vi "FPGA Read Sample.vi"(9 "Number samples\nafter trigger":i32, 10 "Number of Channels":i32, 11 "Timeout":i32) -> (0 "error out":errorcluster, 1 "Different Channel Count":bool, 2 "DMA FIFO Full":bool, 3 "Actual Loop Period (ticks)":u32)   [LabVIEW 2014]
uses:
  <vilib>/rvi/eio/common/nirviEmuClasses.ctl
  <vilib>/rvi/Emulation/niFpgaGetClockAttributes.vi
  <vilib>/rvi/Emulation/niFpgaSctlEmulationGetInTimedLoop.vi
  <vilib>/rvi/Emulation/niFpgaEmulationReportErrorSimple.vi
  FPGA Globals.vi
  <vilib>/rvi/eio/common/nirviEmuTemplateMethod_errors.vi
  <vilib>/rvi/interface/RandomDataEmulation/niFpgaRandomDataHandleErrors.vi
  <vilib>/rvi/Emulation/niFpgaProcessEmulError.vi
  <vilib>/rvi/Emulation/niFpgaCriticalErrorInLSC.vi
  <vilib>/eio/EIOGrowableMethodNode/genericMethod/EIOGrowableMethodNode.xnode
  <vilib>/rvi/eio/nirviEIOMethodImplementation/nirviEIOMethodImplementation.xnode
  <vilib>/rvi/eio/nirviErrorMerge/nirviErrorMerge.xnode
  <vilib>/rvi/DataTransferAndStorage/Container/XNode/niFpgaContainer.xnode
  <vilib>/rvi/interface/RandomDataEmulation/nirviRandomDataFpgaReadWriteTemplate.vi
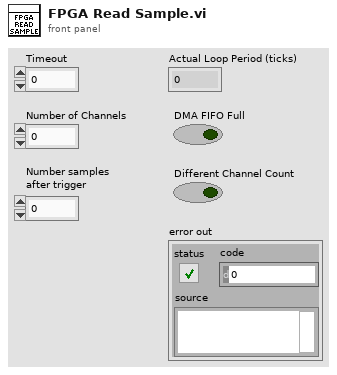
[diagram p1: front panel]
types:
  T1 = typedef "nirviEmuClasses.ctl" = enum16{"IO Read", "IO Write", "Method", "Property Read", "Property Write"}
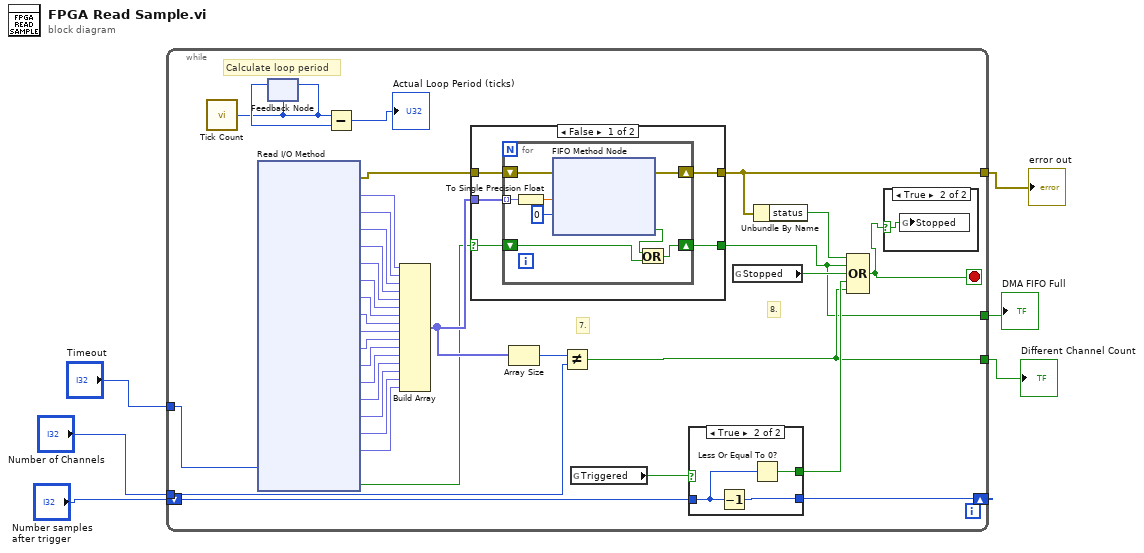
[diagram p0: block diagram]
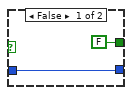
[diagram p3: hidden frame]
diagram:
  n1 = while {
    tunnel: [w41] -> w1
    tunnel: "Number of Channels" -> [w33]
    shift-right: [w30] -> _
    shift-left: "Number samples\nafter trigger" -> [w31]
    tunnel: [w26] -> w4
    tunnel: [w25] -> w5
    tunnel: "Timeout" -> [w23]
    stop <- w29 stop-if-true
    # "Calculate loop period"
    # "8."
    # "7."
    n2 = call "Tick Count"() -> ("Tick Count(Ticks)"=w35:u32)
    n3 = xnode "Read I/O Method"("Timeout"=w23) -> ("error out"=w40:errorcluster, "Mod2/AI0"=w24:fxp<+/-,24,5>, "Mod2/AI1"=w22:fxp<+/-,24,5>, "Mod2/AI2"=w21:fxp<+/-,24,5>, "Mod2/AI3"=w20:fxp<+/-,24,5>, "Mod2/AI4"=w19:fxp<+/-,24,5>, "Mod2/AI5"=w18:fxp<+/-,24,5>, "Mod2/AI6"=w17:fxp<+/-,24,5>, "Mod2/AI7"=w16:fxp<+/-,24,5>, "Mod2/AI8"=w15:fxp<+/-,24,5>, "Mod2/AI9"=w14:fxp<+/-,24,5>, "Mod2/AI10"=w13:fxp<+/-,24,5>, "Mod2/AI11"=w12:fxp<+/-,24,5>, "Mod2/AI12"=w11:fxp<+/-,24,5>, "Mod2/AI13"=w10:fxp<+/-,24,5>, "Mod2/AI14"=w9:fxp<+/-,24,5>, "Mod2/AI15"=w8:fxp<+/-,24,5>, "Timed Out"=w7:bool)  [unwired: 17 in, 16 out]
    n4 = feedback #1(w35) -> (w36:u32)
    n5 = feedback-in #1(w35) -> ()
    n6 = Subtract(x=w35, y=w36) -> (x-y=→"Actual Loop Period (ticks)":u32)
    n7 = Build Array(w24, w22, w21, w20, w19, w18, w17, w16, w15, w14, w13, w12, w11, w10, w9, w8) -> (w37:fxp<+/-,24,5>[])
    n8 = case shown="False" w7 {
      selector: w7 -> [w660 w673]
      tunnel: w37 -> [w664 _]
      tunnel: [w663 w674] -> w41
      tunnel: [w662 w673] -> w25
      tunnel: w40 -> [w661 w674]
      frame False {
        n9 = for {
          tunnel: w664 -> [w670] mode=indexing
          shift-right: [w671] -> w663
          shift-left: w661 -> [w672]
          shift-right: [w668] -> w662
          shift-left: w660 -> [w667]
          n10 = To Single Precision Float(number=w670) -> (single precision float=w666:sgl)
          n11 = xnode ("FIFO Method Node")("Element"=w666, "Timeout"=0, "error in (no error)"=w672) -> ("Timed Out?"=w669:bool, "error out"=w671:errorcluster)  [unwired: 1 in, 1 out]
          n12 = Or(x=w669, y=w667) -> (x .or. y?=w668:bool)
        }
      }
      frame True {
      }
    }
    n13 = Array Size(array=w37) -> (size(s)=w38:i32)
    n14 = Not Equal?(x=w38, y=w33) -> (x != y?=w26:bool)
    n15 = global read "FPGA Globals.vi" "Triggered"() -> (w27:bool)
    n16 = case shown="True" w27 {
      tunnel: [FALSE w658] -> w32
      tunnel: w31 -> [w655 w657]
      tunnel: [w655 w659] -> w30
      frame False {
      }
      frame True {
        n17 = Decrement(x=w657) -> (x-1=w659:i32)
        n18 = Less Or Equal To 0?(x=w657) -> (x <= 0?=w658:bool)
      }
    }
    n19 = global read "FPGA Globals.vi" "Stopped"() -> (w28:bool)
    n20 = Unbundle By Name(w41) -> ("status"=w39:bool)
    n21 = Compound Arithmetic op=OR(w39, w25, w28, w32, w26) -> (w29:bool)
    n22 = case shown="True" w29 {
      selector: w29 -> [_ w654]
      frame False {
      }
      frame True {
        n23 = global write "FPGA Globals.vi" "Stopped"(w654) -> ()
      }
    }
  }
  "DMA FIFO Full" <- w5
  "Different Channel Count" <- w4
  "error out" <- w1
